vi "Generate CPTR.vi"(8 "sync.cptr.adjust":u16, 11 "sync.resources":T1) -> (3 "sync.resources":T1)   [LabVIEW 2013, in "ni579x Synchronization v1 FPGA.lvlib"]
doc: "Generate the CPTR (common periodic time reference)."
uses:
  <instrlib>/ni579x/Synchronization/v1/FPGA/ni579x Synchronization v1 FPGA.lvlib
  <instrlib>/ni579x/Synchronization/v1/FPGA/Implementation/Resources.ctl
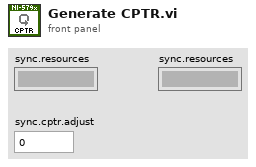
[diagram p1: front panel]
types:
  T1 = typedef "ni579x Synchronization v1 FPGA.lvlib/Resources.ctl" = cluster{"master":refnum<k21>, "meas.enable":refnum<k21>, "meas.ready":refnum<k21>, "meas.arm":refnum<k21>, "meas.valid":refnum<k21>, "meas.value":refnum<k21>, "meas.oversample clock":refnum<k21>, "meas.oversample factor":refnum<k21>, "cptr":refnum<k21>, "cptr.adjust":refnum<k21>, "cptr.period":refnum<k21>}
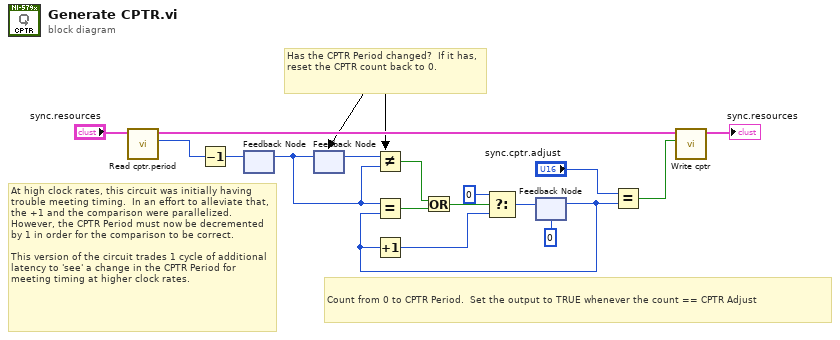
[diagram p0: block diagram]
diagram:
  # "At high clock rates, this circuit was initially having trouble meeting timing.  In an effort to alleviate that, the +1 and the comparison were parallelized.  However, the CPTR Period must now be decremented by 1 in order for the comparison to be correct.  \n\nThis version of the circuit trades 1 cycle of additional latency to 'see' a change in the CPTR Period for meeting timing at higher clock rates."
  # "Has the CPTR Period changed?  If it has, reset the CPTR count back to 0."
  # "Count from 0 to CPTR Period.  Set the output to TRUE whenever the count == CPTR Adjust"
  n1 = call <instrlib>:"Read cptr.period.vi"("sync.resources"="sync.resources") -> ("cptr.period"=w4:u16, "sync.resources"=w9:T1)  [unwired: 9 in]
  n2 = Decrement(x=w4) -> (x-1=w5:u16)
  n3 = feedback #1() -> (w6:u16)  [unwired: 1 in]
  n4 = feedback-in #1(w5) -> ()
  n5 = feedback #2() -> (w14:u16)  [unwired: 1 in]
  n6 = feedback-in #2(w6) -> ()
  n7 = Not Equal?(x=w14, y=w6) -> (x != y?=w17:bool)
  n8 = feedback #3(u16 0) -> (w3:u16)
  n9 = Equal?(x=w6, y=w3) -> (x = y?=w16:bool)
  n10 = Increment(x=w3) -> (x+1=w13:u16)
  n11 = Or(x=w17, y=w16) -> (x .or. y?=w15:bool)
  n12 = Select(t=u16 0, s=w15, f=w13) -> (s? t:f=w12:u16)
  n13 = feedback-in #3(w12) -> ()
  n14 = Equal?(x="sync.cptr.adjust", y=w3) -> (x = y?=w7:bool)
  n15 = call <instrlib>:"Write cptr.vi"("cptr"=w7, "sync.resources"=w9) -> ("sync.resources"=→"sync.resources":T1)  [unwired: 9 in]
